vi "Add Connection to State (SysDef).vi"(8 "error in (no error)":errorcluster, 9 "Connection":T1, 10 "State":string, 11 "Channel Ref in":T2 format="%.0x") -> (0 "error out":errorcluster, 3 "Channel Ref out":T2=18446744073709551615 format="%.0x")   [LabVIEW 2017, in "Switch Scripting.lvlib"]
uses:
  Switch Scripting.lvlib
  <vilib>/NI Veristand/Custom Device API/Custom Device Item Ref.ctl
  Connection.ctl
  NationalInstruments.VeriStand.SystemDefinitionAPI
  <vilib>/NI VeriStand/Custom Device API/Custom Device API.lvlib
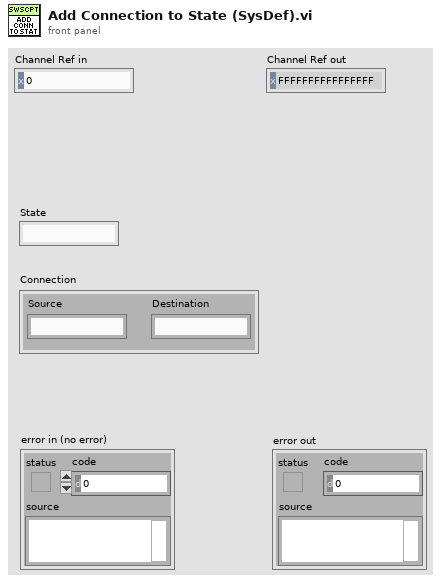
[diagram p1: front panel]
types:
  T1 = typedef "Switch Scripting.lvlib/Connection.ctl" = cluster{"Source":string, "Destination":string}
  T2 = typedef "Custom Device API.lvlib/Custom Device Item Ref.ctl" = u64
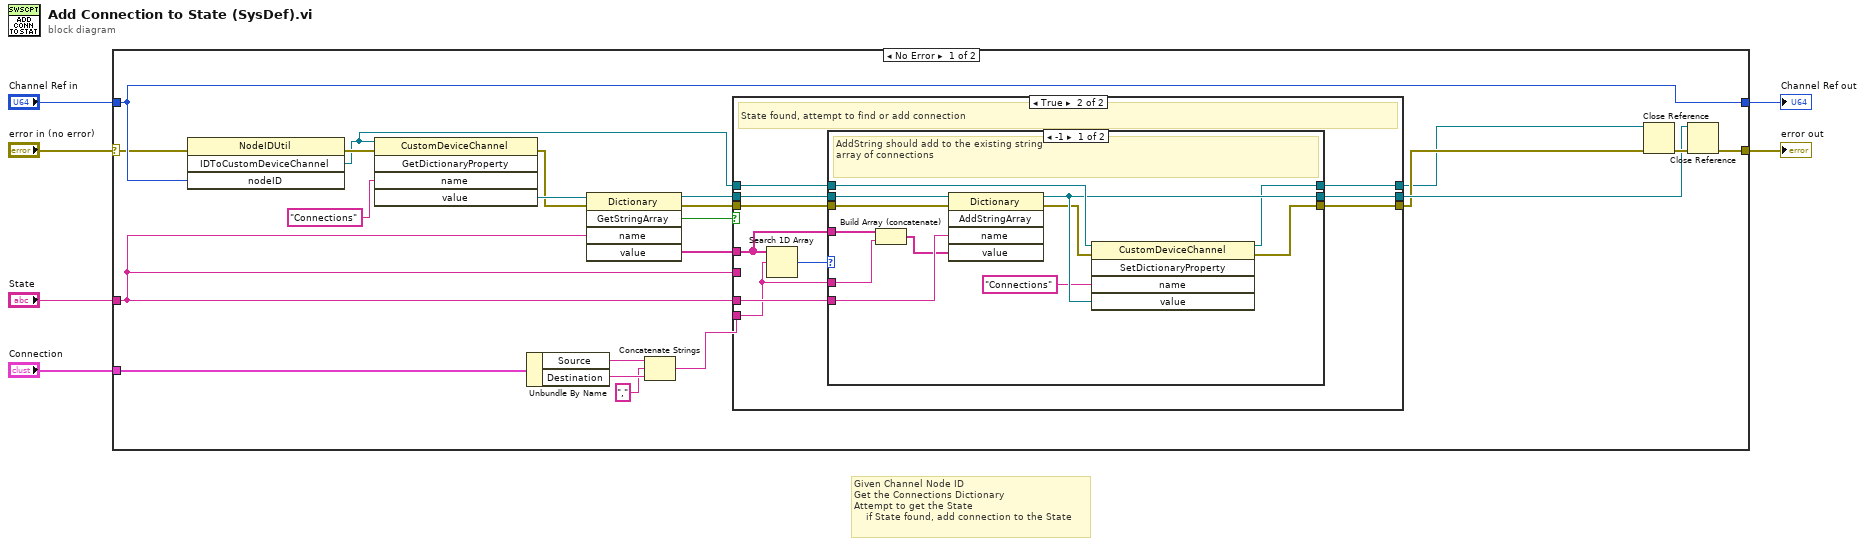
[diagram p0: block diagram]
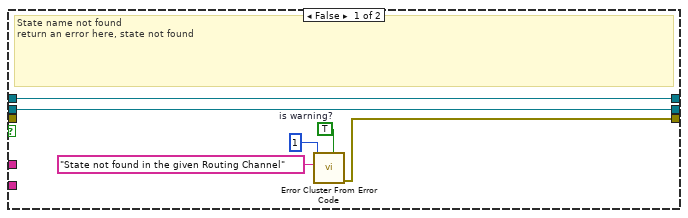
[diagram p2: hidden frame]
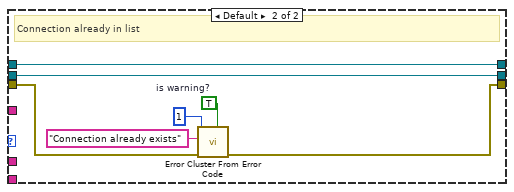
[diagram p3: hidden frame]
diagram:
  # "Given Channel Node ID\nGet the Connections Dictionary\nAttempt to get the State\n    if State found, add connection to the State"
  n1 = case shown="No Error" "error in (no error)" {
    selector: "error in (no error)" -> [w23 w65]
    tunnel: [w28 w65] -> w5
    tunnel: "Channel Ref in" -> [w24 w64]
    tunnel: [w24 w64] -> w3
    tunnel: "State" -> [w11 _]
    tunnel: "Connection" -> [w18 _]
    frame No Error {
      n2 = invoke class="NodeIDUtil" method="IDToCustomDeviceChannel"(error in=w23, "nodeID"=w24) -> (error out=w26:errorcluster, "IDToCustomDeviceChannel"=w8:refnum<k24>)  [unwired: 2 in, 2 out]
      n3 = invoke class="CustomDeviceChannel" method="GetDictionaryProperty"(reference=w8, error in=w26, "name"="Connections") -> (error out=w20:errorcluster, "value"=w21:refnum<k24>)  [unwired: 2 in, 3 out]
      n4 = Unbundle By Name(w18) -> ("Source"=w15:string, "Destination"=w16:string)
      n5 = invoke class="Dictionary" method="GetStringArray"(reference=w21, error in=w20, "name"=w11) -> (reference out=w12:refnum<k24>, error out=w17:errorcluster, "GetStringArray"=w19:bool, "value"=w22:string[])  [unwired: 2 in, 1 out]
      n6 = Concatenate Strings(w15, "," ("string"), w16) -> (w13:string)
      n7 = case shown="True" w19 {
        tunnel: w22 -> [_ w36]
        tunnel: w17 -> [_ w43]
        tunnel: w13 -> [_ w35]
        tunnel: [w31 w42] -> w9
        tunnel: w11 -> [_ w41]
        tunnel: w12 -> [w30 w40]
        tunnel: [w30 w39] -> w10
        tunnel: w11 -> [_ _]
        tunnel: w8 -> [w29 w38]
        tunnel: [w29 w37] -> w7
        frame False {
          w33 = TRUE  # is warning?
          # "State name not found\nreturn an error here, state not found"
          n8 = call <vilib>:"Error Cluster From Error Code.vi"("is warning? (False)"=w33, "error message (\"\")"="State not found in the given Routing Channel" ("error message (\"\")"), "error code (0)"=1) -> ("error out"=w31:errorcluster)  [unwired: 6 in]
        }
        frame True {
          # "State found, attempt to find or add connection"
          n9 = Search 1D Array(1D array=w36, element=w35) -> (index of element=w44:i32)  [unwired: 1 in]
          n10 = case shown="-1" w44 {
            tunnel: w43 -> [w54 w60]
            tunnel: [w49 w59] -> w42
            tunnel: w41 -> [w56 _]
            tunnel: w40 -> [w55 w58]
            tunnel: [w52 w58] -> w39
            tunnel: w38 -> [w53 w57]
            tunnel: [w48 w57] -> w37
            tunnel: w36 -> [w47 _]
            tunnel: w35 -> [w46 _]
            frame -1 {
              # "AddString should add to the existing string\narray of connections"
              n11 = Build Array (concatenate)(w47, w46) -> (w45:string[])
              n12 = invoke class="Dictionary" method="AddStringArray"(reference=w55, error in=w54, "name"=w56, "value"=w45) -> (reference out=w52:refnum<k24>, error out=w50:errorcluster)  [unwired: 1 in, 3 out]
              n13 = invoke class="CustomDeviceChannel" method="SetDictionaryProperty"(reference=w53, error in=w50, "name"="Connections", "value"=w52) -> (reference out=w48:refnum<k24>, error out=w49:errorcluster)  [unwired: 1 in, 3 out]
            }
            frame Default {
              w62 = TRUE  # is warning?
              # "Connection already in list"
              n14 = call <vilib>:"Error Cluster From Error Code.vi"("is warning? (False)"=w62, "error in (no error)"=w60, "error message (\"\")"="Connection already exists" ("error message (\"\")"), "error code (0)"=1) -> ("error out"=w59:errorcluster)  [unwired: 5 in]
            }
          }
        }
      }
      n15 = Close Reference(reference=w7, error in (no error)=w9) -> (error out=w27:errorcluster)
      n16 = Close Reference(reference=w10, error in (no error)=w27) -> (error out=w28:errorcluster)
    }
    frame Error {
    }
  }
  "Channel Ref out" <- w3
  "error out" <- w5
